vi "Clear All Discretes.vi"(8 "error in":errorcluster, 11 "SL_SC in":refnum<class "SL_SC.lvclass">) -> (0 "error out":errorcluster, 3 "SL_SC out":refnum<class "SL_SC.lvclass">)   [LabVIEW 2019, in "SL_SC.lvlib" / "SL_SC.lvclass"]
uses:
  Library/SL_SC.lvclass
  builds/Instruments/DIG_IO.lvlibp/Library/DIG_IO.lvclass
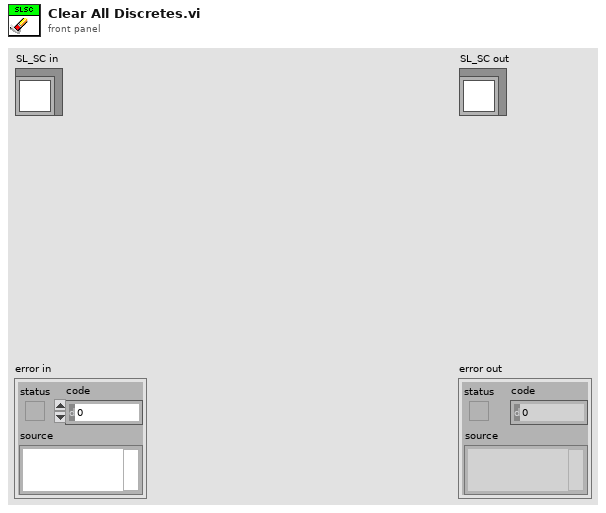
[diagram p1: front panel]
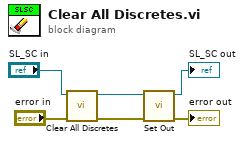
[diagram p0: block diagram]
diagram:
  n1 = call-parent "Clear All Discretes.vi"("error in"="error in", "DIG_IO in"="SL_SC in") -> ("error out"=w3:errorcluster, "DIG_IO out"=w4:refnum<class "SL_SC.lvclass">)  [unwired: 8 in]
  n2 = call-dynamic "Set Out.vi"("error in"=w3, "SL_SC in"=w4) -> ("error out"=→"error out":errorcluster, "SL_SC out"=→"SL_SC out":refnum<class "SL_SC.lvclass">)  [unwired: 8 in]
